vi "GenNet Receive Message.vi"(6 "timeout [ms]":i32=1000, 8 "error in (no error)":errorcluster, 11 "TCP Network Connection in":refnum<k5>) -> (0 "error out":errorcluster, 2 "Message Data":variant, 3 "TCP Network Connection out":refnum<k5>)   [LabVIEW 2014, in "hse-gennet.lvlib"]
doc: "Receives a message sent by a GenNet-Client module. The first 4 bytes of the message contain the lenght of the actual data sent. The received message is converted to a variant.\n\n____\nHAMPEL SOFTWARE ENGINEERING v0.7.0 (2018-07-16 18:12)"
uses:
  hse-gennet.lvlib
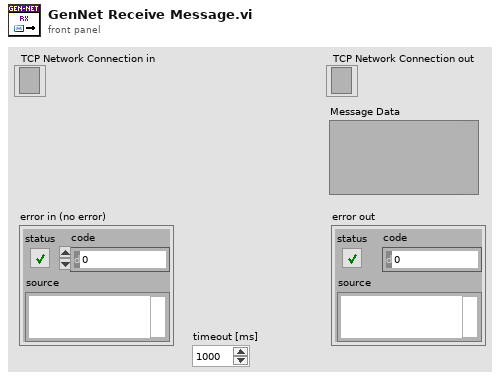
[diagram p1: front panel]
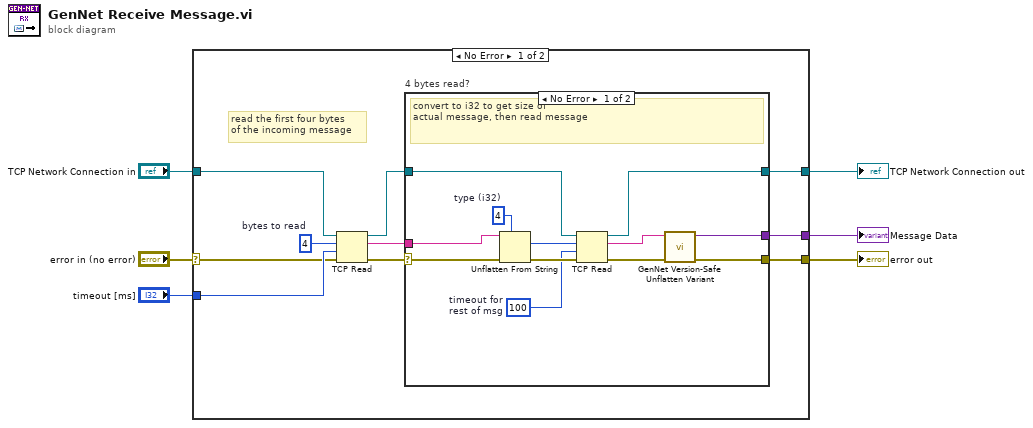
[diagram p0: block diagram]
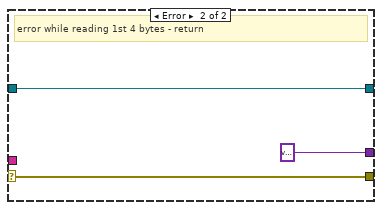
[diagram p2: hidden frame]
diagram:
  n1 = case shown="No Error" "error in (no error)" {
    selector: "error in (no error)" -> [w7 w32]
    tunnel: "TCP Network Connection in" -> [w15 w33]
    tunnel: [w14 w33] -> w5
    tunnel: "timeout [ms]" -> [w11 _]
    tunnel: [w10 w32] -> w3
    tunnel: [w9 _] -> w2
    frame No Error {
      w16 = 4  # bytes to read
      # "read the first four bytes\nof the incoming message"
      n2 = TCP Read(connection ID=w15, bytes to read=w16, error in (no error)=w7, 9:w11) -> (connection ID out=w12:refnum<k5>, data out=w13:string, error out=w8:errorcluster)  [unwired: 1 in]
      n3 = case "4 bytes read?" shown="No Error" w8 {
        selector: w8 -> [w21 w30]
        tunnel: [w28 w31] -> w14
        tunnel: w13 -> [w27 _]
        tunnel: w12 -> [w23 w31]
        tunnel: [w19 w30] -> w10
        tunnel: [w18 variant] -> w9
        frame No Error {
          w26 = 4  # type (i32)
          w22 = 100  # timeout for  rest of msg
          # "convert to i32 to get size of\nactual message, then read message"
          n4 = Unflatten From String(type=w26, binary string=w27, error in (no error)=w21) -> (value=w25:i32, error out=w24:errorcluster)  [unwired: 2 in, 1 out]
          n5 = TCP Read(connection ID=w23, bytes to read=w25, error in (no error)=w24, 9:w22) -> (connection ID out=w28:refnum<k5>, data out=w17:string, error out=w20:errorcluster)  [unwired: 1 in]
          n6 = call "GenNet Version-Safe Unflatten Variant.vi"("error in"=w20, "Flattened Data"=w17) -> ("error out"=w19:errorcluster, "Message Data"=w18:variant)  [unwired: 8 in]
        }
        frame Error {
          # "error while reading 1st 4 bytes - return"
        }
      }
    }
    frame Error {
    }
  }
  "error out" <- w3
  "TCP Network Connection out" <- w5
  "Message Data" <- w2
